vi "Update Item.vi"(8 "error in (no error)":errorcluster, 10 "All Data":refnum<class "Data Item.lvclass">[](array[class]), 11 "Data Item in":refnum<class "Data Item.lvclass">) -> (0 "error out":errorcluster, 2 "All Data out":refnum<class "Data Item.lvclass">[](array[class]), 3 "Data Item out":refnum<class "Data Item.lvclass">)   [LabVIEW 2026, in "VILab.lvlib" / "Data Item.lvclass"]
uses:
  Data Item.lvclass
  VILab.lvlib
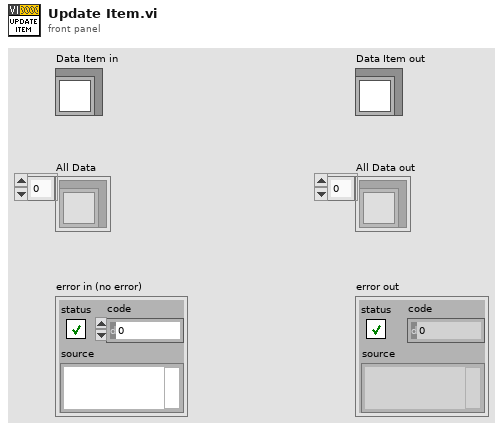
[diagram p1: front panel]
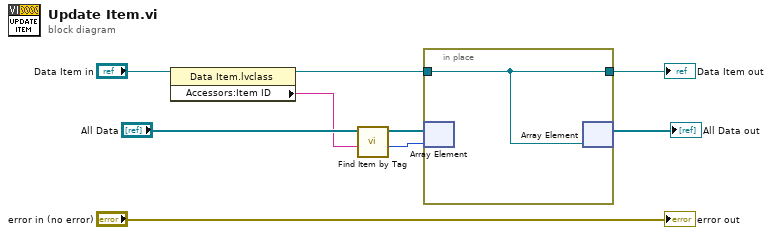
[diagram p0: block diagram]
diagram:
  n1 = property class="Data Item.lvclass"(reference="Data Item in") -> (reference out=w3:refnum<class "Data Item.lvclass">, "Accessors:Item ID"=w7:string)  [unwired: 1 in, 1 out]
  n2 = call "Find Item by Tag.vi"("Tree Tag"=w7, "All Data"="All Data") -> ("Index"=w4:i32, "All Data out"=w5:refnum<class "Data Item.lvclass">[])  [unwired: 7 in, 1 out]
  n3 = in-place {
    in-place-border: w3 -> [w10]
    in-place-border: [w10] -> w2
    n4 = in-place-array #1(w5, w4) -> ()  [unwired: 1 out]
    n5 = in-place-array #1(w10) -> (→"All Data out":refnum<class "Data Item.lvclass">[])  [unwired: 1 out]
  }
  "Data Item out" <- w2
  "error out" <- "error in (no error)"
